vi "sub 2.vi"(6 "Current Missing Points":i32, 9 "Previous Producer Iterations":i32, 10 "Producer Iterations":i32, 11 "Current Duplicated Points":i32) -> (2 "Update Missing Points":i32, 3 "Updated Duplicated Points":i32)   [LabVIEW 2015]
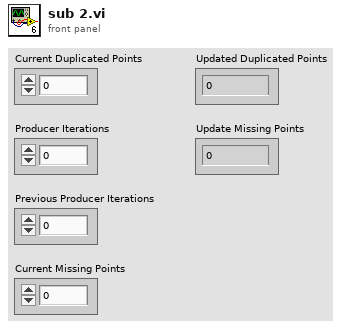
[diagram p1: front panel]
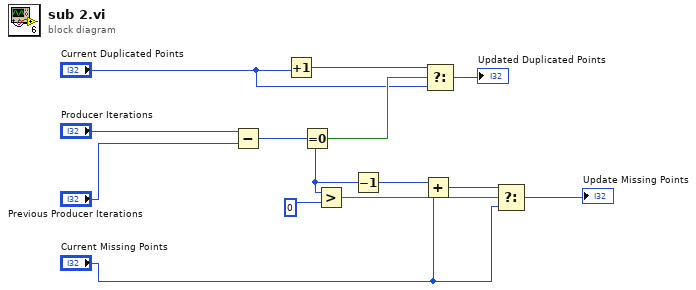
[diagram p0: block diagram]
diagram:
  n1 = Subtract(x="Producer Iterations", y="Previous Producer Iterations") -> (x-y=w6:i32)
  n2 = Increment(x="Current Duplicated Points") -> (x+1=w1:i32)
  n3 = Equal To 0?(x=w6) -> (x = 0?=w5:bool)
  n4 = Greater?(x=w6, y=0) -> (0:w9:bool)
  n5 = Decrement(x=w6) -> (x-1=w8:i32)
  n6 = Add(x=w8, y="Current Missing Points") -> (x+y=w10:i32)
  n7 = Select(t=w1, s=w5, f="Current Duplicated Points") -> (s? t:f=→"Updated Duplicated Points":i32)
  n8 = Select(t=w10, s=w9, f="Current Missing Points") -> (s? t:f=→"Update Missing Points":i32)
